vi "Read Read Write.vi"(8 "error in (no error)":errorcluster, 11 "IO in":refnum<class "IO.lvclass">) -> (0 "error out":errorcluster, 2 "R/W":bool, 3 "IO out":refnum<class "IO.lvclass">)   [LabVIEW 2021, in "IO.lvclass"]
uses:
  IO.lvclass
  IO.lvclass/IO.ctl
  <vilib>/DAQmx/read.llb/DAQmx Read (Digital Bool 1Line 1Point).vi
  <vilib>/DAQmx/miscellaneous.llb/DAQmx Fill In Error Info.vi
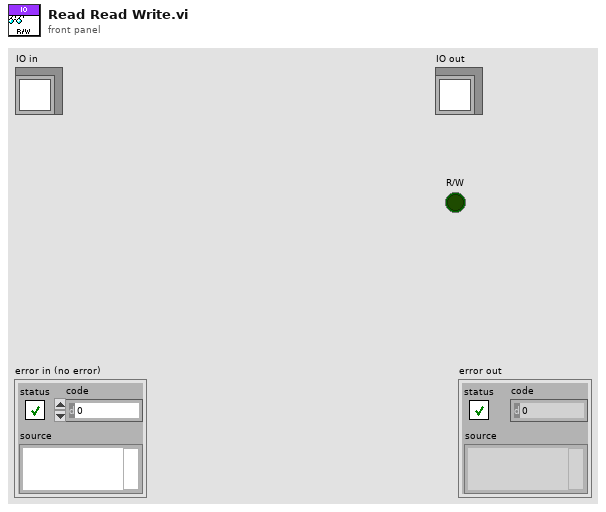
[diagram p1: front panel]
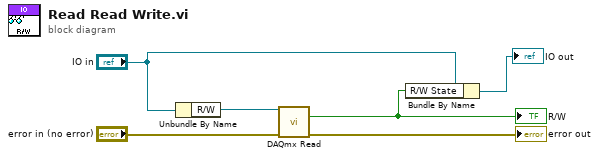
[diagram p0: block diagram]
diagram:
  n1 = Unbundle By Name("IO in") -> ("R/W"=w4:refnum<k21>)
  n2 = call-poly <vilib>:"DAQmx Read.vi"("task/channels in"=w4, "error in"="error in (no error)") -> ("data"=w2:bool, "error out"=→"error out":errorcluster)  [unwired: 11 in, 1 out]
  "R/W" <- w2
  n3 = Bundle By Name(cluster="IO in", "R/W State"=w2) -> (→"IO out":refnum<class "IO.lvclass">)
